vi "test_syncAveraging.vi"() -> ()   [LabVIEW 2016]
uses:
  <vilib>/rvi/DesktopExecutionNode/Execution/niFpgaDEN_Execute.vi
  <vilib>/rvi/DesktopExecutionNode/DesktopExecutionNode.xnode
panel:
  out "dataIn":dbl[](graph)
  out "Array":T1(array[cluster])
  in  "numTicks":i32
types:
  T1 = cluster{"waveMaxAvg":fxp<+/-,24,16>, "outputValid":bool}[]
  T2 = cluster{"waveMaxAvg":fxp<+/-,24,16>, "outputValid":bool}
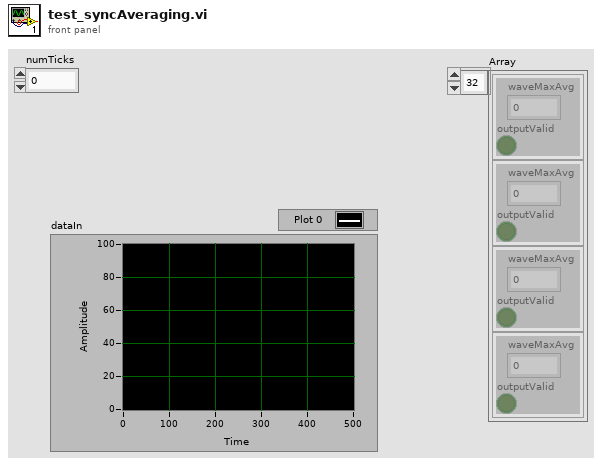
[diagram p1: front panel]
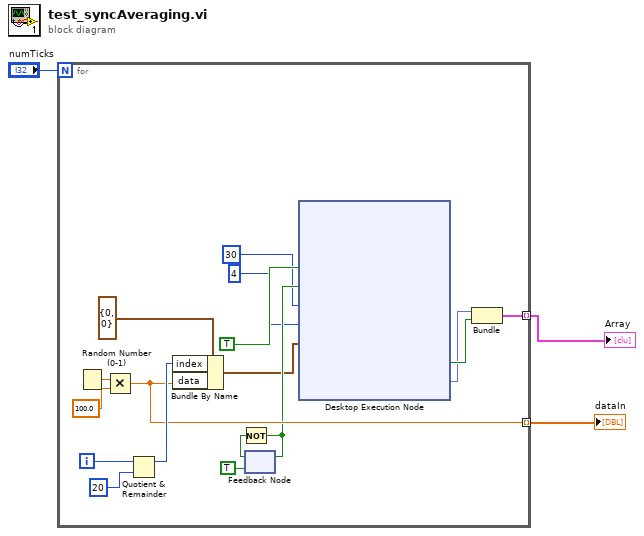
[diagram p0: block diagram]
diagram:
  n1 = for {
    N: "numTicks" -> [_]
    tunnel: [w12] -> w1 mode=indexing
    tunnel: [w11] -> w2 mode=indexing
    i -> [w17]
    n2 = Random Number (0-1)() -> (number: 0 to 1=w19:dbl)
    n3 = Multiply(x=w19, y=100.0) -> (x*y=w11:dbl)
    n4 = Quotient & Remainder(x=w17, y=20) -> (x-y*floor(x/y)=w16:i32)  [unwired: 1 out]
    n5 = Bundle By Name(cluster=cluster{"index":u16, "data":i16} {"index"=0, "data"=0} ("input"), "index"=w16, "data"=w11) -> (w6:cluster{"index":u16, "data":i16})
    n6 = feedback #1(TRUE) -> (w14:bool)
    n7 = Not(x=w14) -> (.not. x?=w10:bool)
    n8 = feedback-in #1(w10) -> ()
    n9 = xnode "Desktop Execution Node"("enable"=TRUE, "inputValid"=w10, "syncPoint"=u16 30, "syncAverageBand"=u16 4, "input"=w6) -> ("outputValid"=w8:bool, "waveMaxAvg"=w7:fxp<+/-,24,16>)  [unwired: 1 in, 1 out]
    n10 = Bundle("waveMaxAvg"=w7, "outputValid"=w8) -> (w12:T2)  [unwired: 1 in]
  }
  "Array" <- w1
  "dataIn" <- w2
